vi "Support_MergeResult.vi"(2 "Results in":T1[](array[typedef]) {"MeasurementValue" format="%.2f"}, 3 "Results in 2":T1[](array[typedef]) {"MeasurementValue" format="%.2f"}, 4 "Results in 3":T1[](array[typedef]) {"MeasurementValue" format="%.2f"}, 5 "Results in 4":T1[](array[typedef]) {"MeasurementValue" format="%.2f"}) -> (16 "Results out":T1[](array[typedef]) {"MeasurementValue" format="%.2f"})   [LabVIEW 2009]
doc: "Merges results."
uses:
  Support_ResultType.ctl
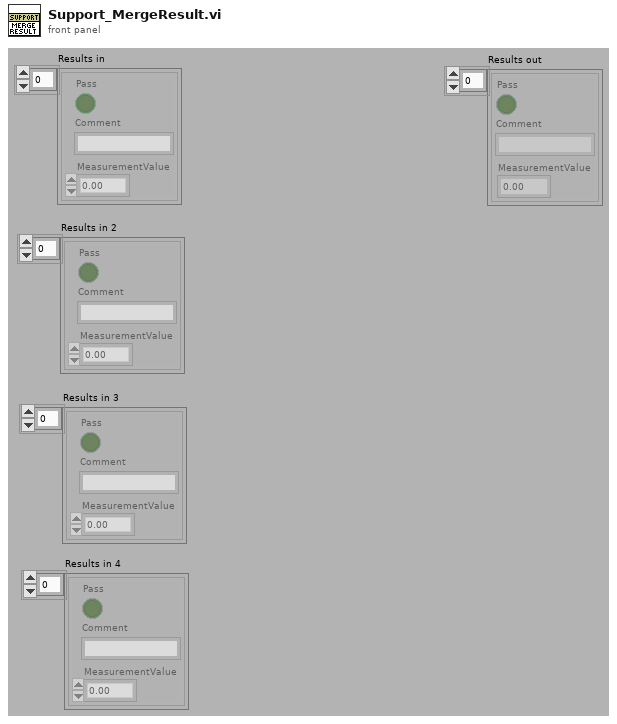
[diagram p1: front panel]
types:
  T1 = typedef "Support_ResultType.ctl" = cluster{"Pass":bool, "Comment":string, "MeasurementValue":dbl}
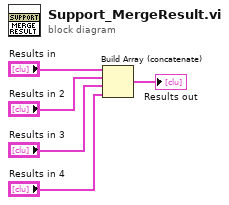
[diagram p0: block diagram]
diagram:
  n1 = Build Array (concatenate)("Results in", "Results in 2", "Results in 3", "Results in 4") -> (→"Results out":T1[])
